vi "Build.vi"(6 "Version":T2, 7 "Build Events":refnum<class "Build Events API.lvclass">, 8 "error in (no error)":errorcluster, 10 "Build Info":T1, 11 "Package Build in":refnum<class "Package Build.lvclass">) -> (0 "error out":errorcluster)   [LabVIEW 2020, in "Builder Tools.lvlib" / "Package Build.lvclass"]
uses:
  Package Build.lvclass
  Builder Core/Version.ctl
  Build Events API/Build Events API.lvclass
  Build Info.ctl
  <vilib>/AppBuilder/AB_API_Simple/Set Build Specification Version (path).vi
  Package Build.lvclass/Package Build.ctl
  <vilib>/AppBuilder/AB_API_Simple/Build (path).vi
  <vilib>/AppBuilder/AB_API_Simple/NI_App_Builder_API.lvlib
  Builder Core/Builder Core.lvlib
  Builder Tools.lvlib
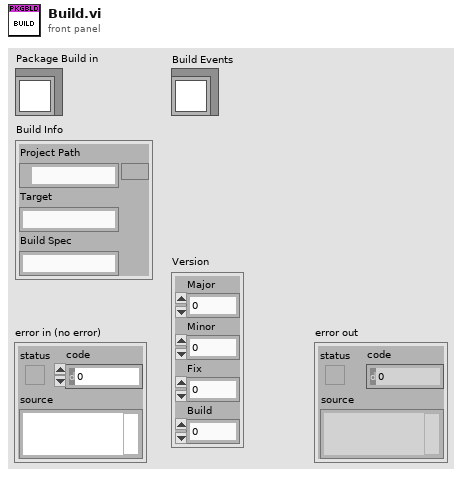
[diagram p1: front panel]
types:
  T1 = typedef "Builder Tools.lvlib/Build Info.ctl" = cluster{"Project Path":path, "Target":string, "Build Spec":string}
  T2 = typedef "Builder Core.lvlib/Version.ctl" = cluster{"Major":u16, "Minor":u16, "Fix":u16, "Build":u16}
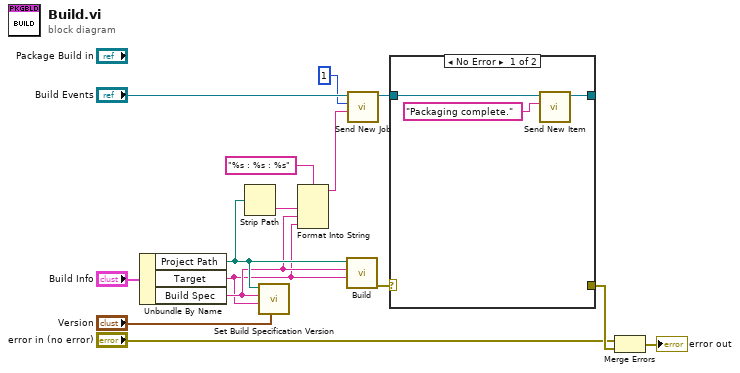
[diagram p0: block diagram]
diagram:
  n1 = Unbundle By Name("Build Info") -> ("Project Path"=w8:path, "Target"=w5:string, "Build Spec"=w6:string)
  n2 = Strip Path(path=w8) -> (name=w7:string)  [unwired: 1 out]
  n3 = call-poly <vilib>:"Set Build Specification Version.vi"("Build Specification Version"="Version", "Name of target (My Computer)"=w5, "Name of build specification"=w6, "Path to project"=w8) -> ()  [unwired: 7 in, 1 out]
  n4 = Format Into String(format string="%s : %s : %s", w7, w6, w5) -> (resulting string=w2:string)  [unwired: 2 in, 1 out]
  n5 = call-poly <vilib>:"Build.vi"("Name of target (My Computer)"=w5, "Name of build specification (if empty: build all)"=w6, "Path to project"=w8) -> ("error out"=w13:errorcluster)  [unwired: 7 in, 1 out]
  n6 = call "Send New Job.vi"("Build"=w2, "Max Progress"=1, "Build Events API in"="Build Events") -> ("Build Events API out"=w3:refnum<class "Build Events API.lvclass">)  [unwired: 7 in, 1 out]
  n7 = case shown="No Error" w13 {
    selector: w13 -> [_ w19]
    tunnel: w3 -> [w18 w20]
    tunnel: [w16 w20] -> _
    tunnel: [_ w19] -> w12
    frame No Error {
      n8 = call "Send New Item.vi"("Message"="Packaging complete.", "Build Events API in"=w18) -> ("Build Events API out"=w16:refnum<class "Build Events API.lvclass">)  [unwired: 8 in, 1 out]
    }
    frame Error {
    }
  }
  n9 = Merge Errors("error in (no error)", w12) -> (→"error out":errorcluster)
